vi "Server - Error Handler.vi"(7 "Component":string="Archive", 8 "error in (no error)":errorcluster, 11 "Message Queue":refnum<queue>) -> (0 "error out":errorcluster)   [LabVIEW 2024]
doc: "Handles errors in the server."
uses:
  Support/Shared/Message Queue/Message Cluster.ctl
  Support/Shared/Message Queue.lvlib
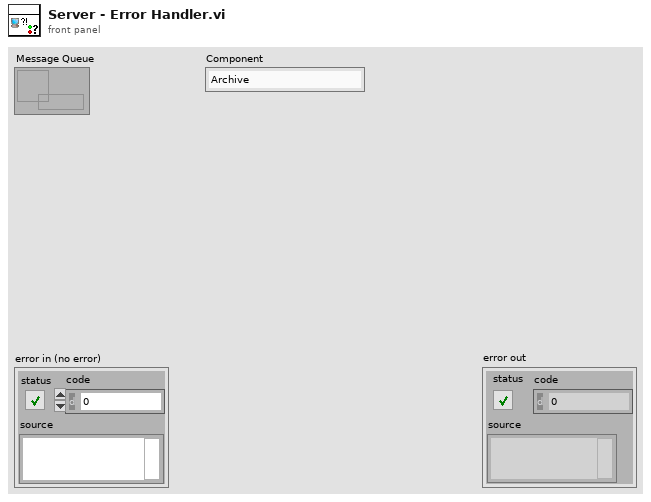
[diagram p1: front panel]
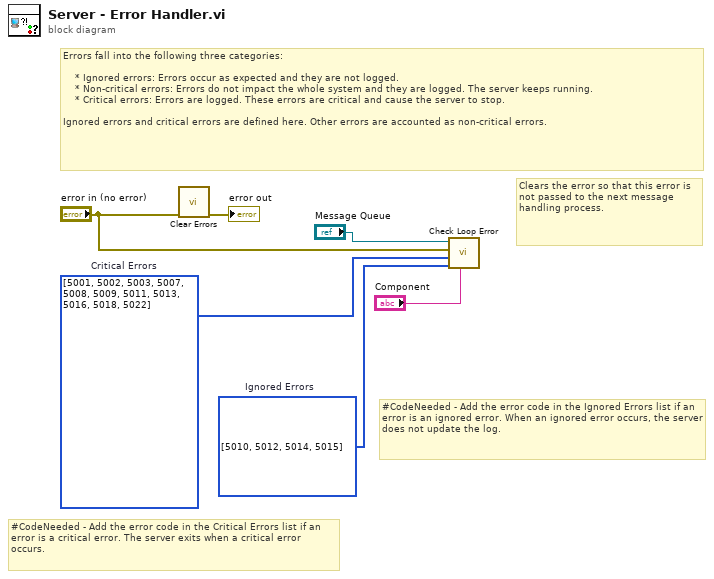
[diagram p0: block diagram]
diagram:
  w2 = i32[] [5010, 5012, 5014, 5015]  # Ignored Errors
  w6 = i32[] [5001, 5002, 5003, 5007, 5008, 5009, 5011, 5013, 5016, 5018, 5022]  # Critical Errors
  # "#CodeNeeded - Add the error code in the Ignored Errors list if an error is an ignored error. When an ignored error occurs, the server does not update the log."
  # "#CodeNeeded - Add the error code in the Critical Errors list if an error is a critical error. The server exits when a critical error occurs."
  # "Errors fall into the following three categories:\n\t \n  \t\t* Ignored errors: Errors occur as expected and they are not logged. \n  \t\t* Non-critical errors: Errors do not impact the whole system and they are logged. The server keeps running.\n\t\t  * Critical errors: Errors are logged. These errors are critical and cause the server to stop.\n\nIgnored errors and critical errors are defined here. Other errors are accounted as non-critical errors."
  # "Clears the error so that this error is not passed to the next message handling process."
  n1 = call <vilib>:"Clear Errors.vi"("error in (no error)"="error in (no error)") -> ("error out"=→"error out":errorcluster)  [unwired: 5 in, 1 out]
  n2 = call "Check Loop Error.vi"("Component"="Component", "Ignored Errors"=w2, "Critical Errors"=w6, "Error to Handle"="error in (no error)", "Message Queue"="Message Queue") -> ()  [unwired: 7 in]
